vi "U3 Multiple IO Example Loop.vi"() -> ()   [LabVIEW 2021]
panel:
  in  "Interval (ms)":u32=500
  in  "stop":bool
  out "FIO5":bool
  out "FIO4":bool
  out "AIN3":dbl format="%.6f"
  out "AIN2":dbl format="%.6f"
  out "AIN1":dbl format="%.6f"
  out "AIN0":dbl format="%.6f"
  in  "FIO7":bool
  in  "FIO6":bool
  in  "DAC0":dbl format="%.4f"
  out "Error Message":string
  out "error out":errorcluster
  # "Outputs DAC0 and FIO6-FIO7.  Aquires AIN0-AIN3 and FIO4-FIO5.  This example\ndoes the proper pin configuration also.  Uses USB on the first found U3."
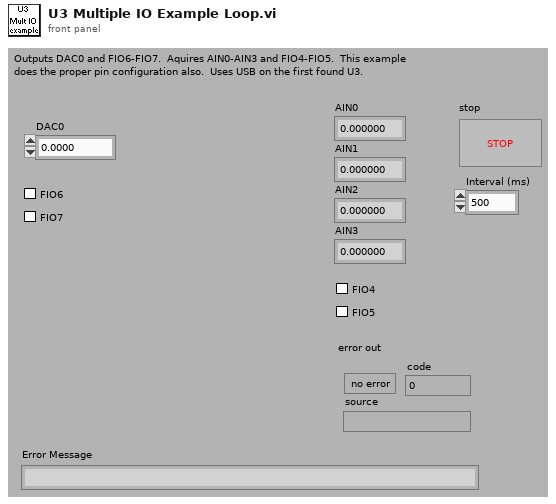
[diagram p1: front panel]
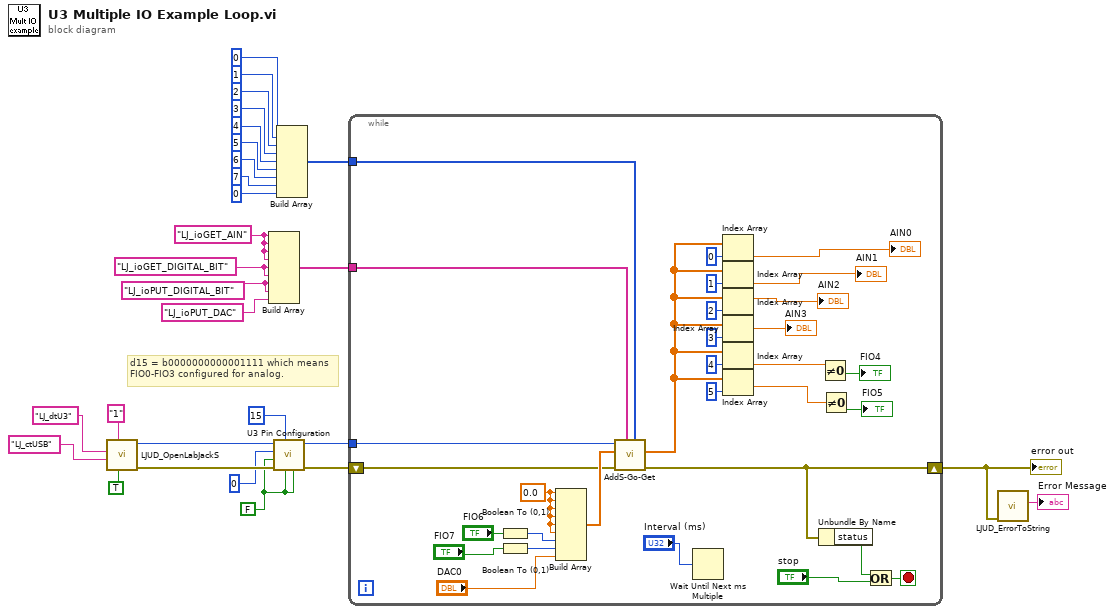
[diagram p0: block diagram]
diagram:
  w1 = FALSE ("Enable DAC1")
  w25 = "LJ_ioPUT_DIGITAL_BIT" ("IOType")
  w27 = "LJ_ioGET_AIN" ("IOType")
  w26 = "LJ_ioGET_DIGITAL_BIT" ("IOType")
  # "d15 = b0000000000001111 which means\nFIO0-FIO3 configured for analog."
  n1 = call "LJUD_OpenLabJackS.vi"("FirstFound"=TRUE, "Address"="1", "ConnectionType"="LJ_ctUSB", "DeviceType"="LJ_dtU3") -> ("error out"=w6:errorcluster, "Handle"=w4:i32)  [unwired: 5 in, 1 out]
  n2 = Build Array(w27, w27, w27, w27, w26, w26, w25, w25, "LJ_ioPUT_DAC" ("IOType")) -> (w24:string[])
  n3 = call "U3 Pin Configuration.vi"("Enable Counter1"=w1, "Enable Counter0"=w1, "FIO/EIO Analog Enable"=15, "error in"=w6, "Enable DAC1"=w1, "Number of Timers Enabled"=u8 0, "Handle In"=w4) -> ("error out"=w7:errorcluster, "Handle Out"=w5:i32)  [unwired: 3 in]
  n4 = Build Array(0, 1, 2, 3, 4, 5, 6, 7, 0) -> (w23:i32[])
  n5 = while {
    shift-left: w7 -> [w31]
    shift-right: [w30] -> w8
    tunnel: w5 -> [w35]
    tunnel: w23 -> [w58]
    tunnel: w24 -> [w59]
    stop <- w34 stop-if-true
    w57 = 0.0 ("Input Element")
    n6 = Boolean To (0,1)(Boolean="FIO6") -> (0, 1=w56:i16)
    n7 = Boolean To (0,1)(Boolean="FIO7") -> (0, 1=w55:i16)
    n8 = Build Array(w57, w57, w57, w57, w57, w57, w56, w55, "DAC0") -> (w54:dbl[])
    n9 = call "AddS-Go-Get.vi"("Channels"=w58, "IOTypes"=w59, "error in"=w31, "Values Write"=w54, "Handle In"=w35) -> ("error out"=w30:errorcluster, "Values Read"=w48:dbl[])  [unwired: 4 in, 1 out]
    n10 = Wait Until Next ms Multiple(millisecond multiple="Interval (ms)") -> ()  [unwired: 1 out]
    n11 = Index Array(array=w48, index=0 ("Index")) -> (element=→"AIN0":dbl)
    n12 = Index Array(array=w48, index=1 ("Index")) -> (element=→"AIN1":dbl)
    n13 = Index Array(array=w48, index=2 ("Index")) -> (element=→"AIN2":dbl)
    n14 = Index Array(array=w48, index=3 ("Index")) -> (element=→"AIN3":dbl)
    n15 = Index Array(array=w48, index=4 ("Index")) -> (element=w46:dbl)
    n16 = Index Array(array=w48, index=5 ("Index")) -> (element=w45:dbl)
    n17 = Unbundle By Name(w30) -> ("status"=w32:bool)
    n18 = Not Equal To 0?(x=w46) -> (x != 0?=→"FIO4":bool)
    n19 = Not Equal To 0?(x=w45) -> (x != 0?=→"FIO5":bool)
    n20 = Or(x=w32, y="stop") -> (x .or. y?=w34:bool)
  }
  "error out" <- w8
  n21 = call "LJUD_ErrorToString.vi"("error in"=w8) -> ("String"=→"Error Message":string)  [unwired: 10 in]
